vi "TestProgram1Keithley2.vi"() -> ()   [LabVIEW 2014]
panel:
  out "Resistance":dbl
  in  "Delay":dbl
  in  "Average Measurements":dbl
  in  "Clear graph?":bool
  out "Resistance VS Temperature":cluster{dbl[], dbl[]}(graph)
  out "Byte Stream File Refnum":refnum<file>
  in  "file path (use dialog)":path
  out "Current Temperature":string
  out "Return":string
  in  "Set Temperature Command":string
  in  "Set Temperature":bool
  out "Return Value Temp":string
  in  "Command Temp":string
  in  "Temp":refnum<visa-resource-name>
  in  "Multimeter 1":refnum<visa-resource-name>
  in  "Measure":bool
  in  "stop":bool
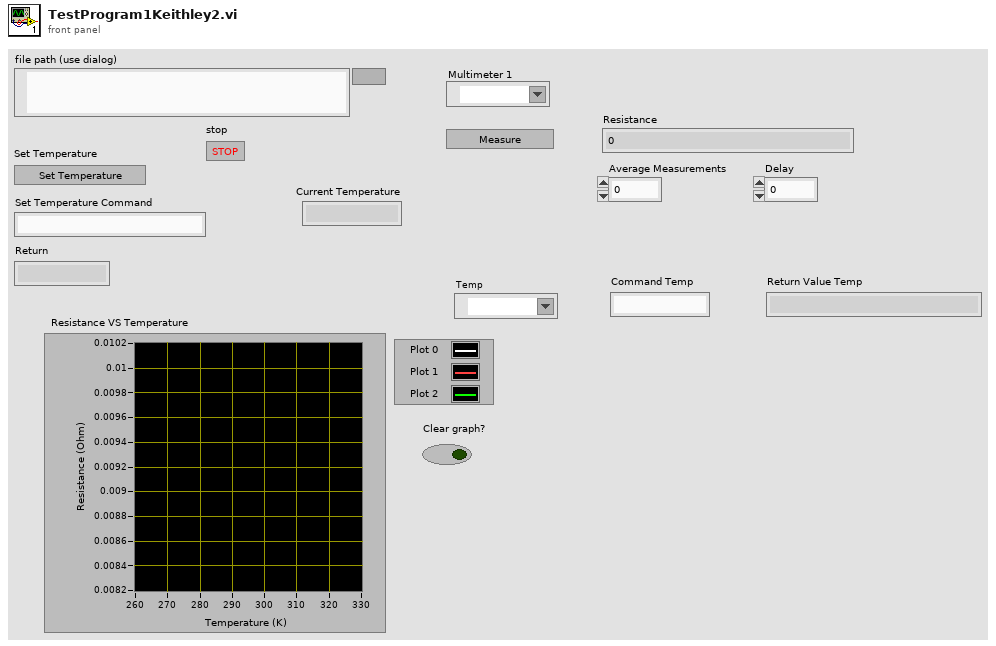
[diagram p1: front panel]
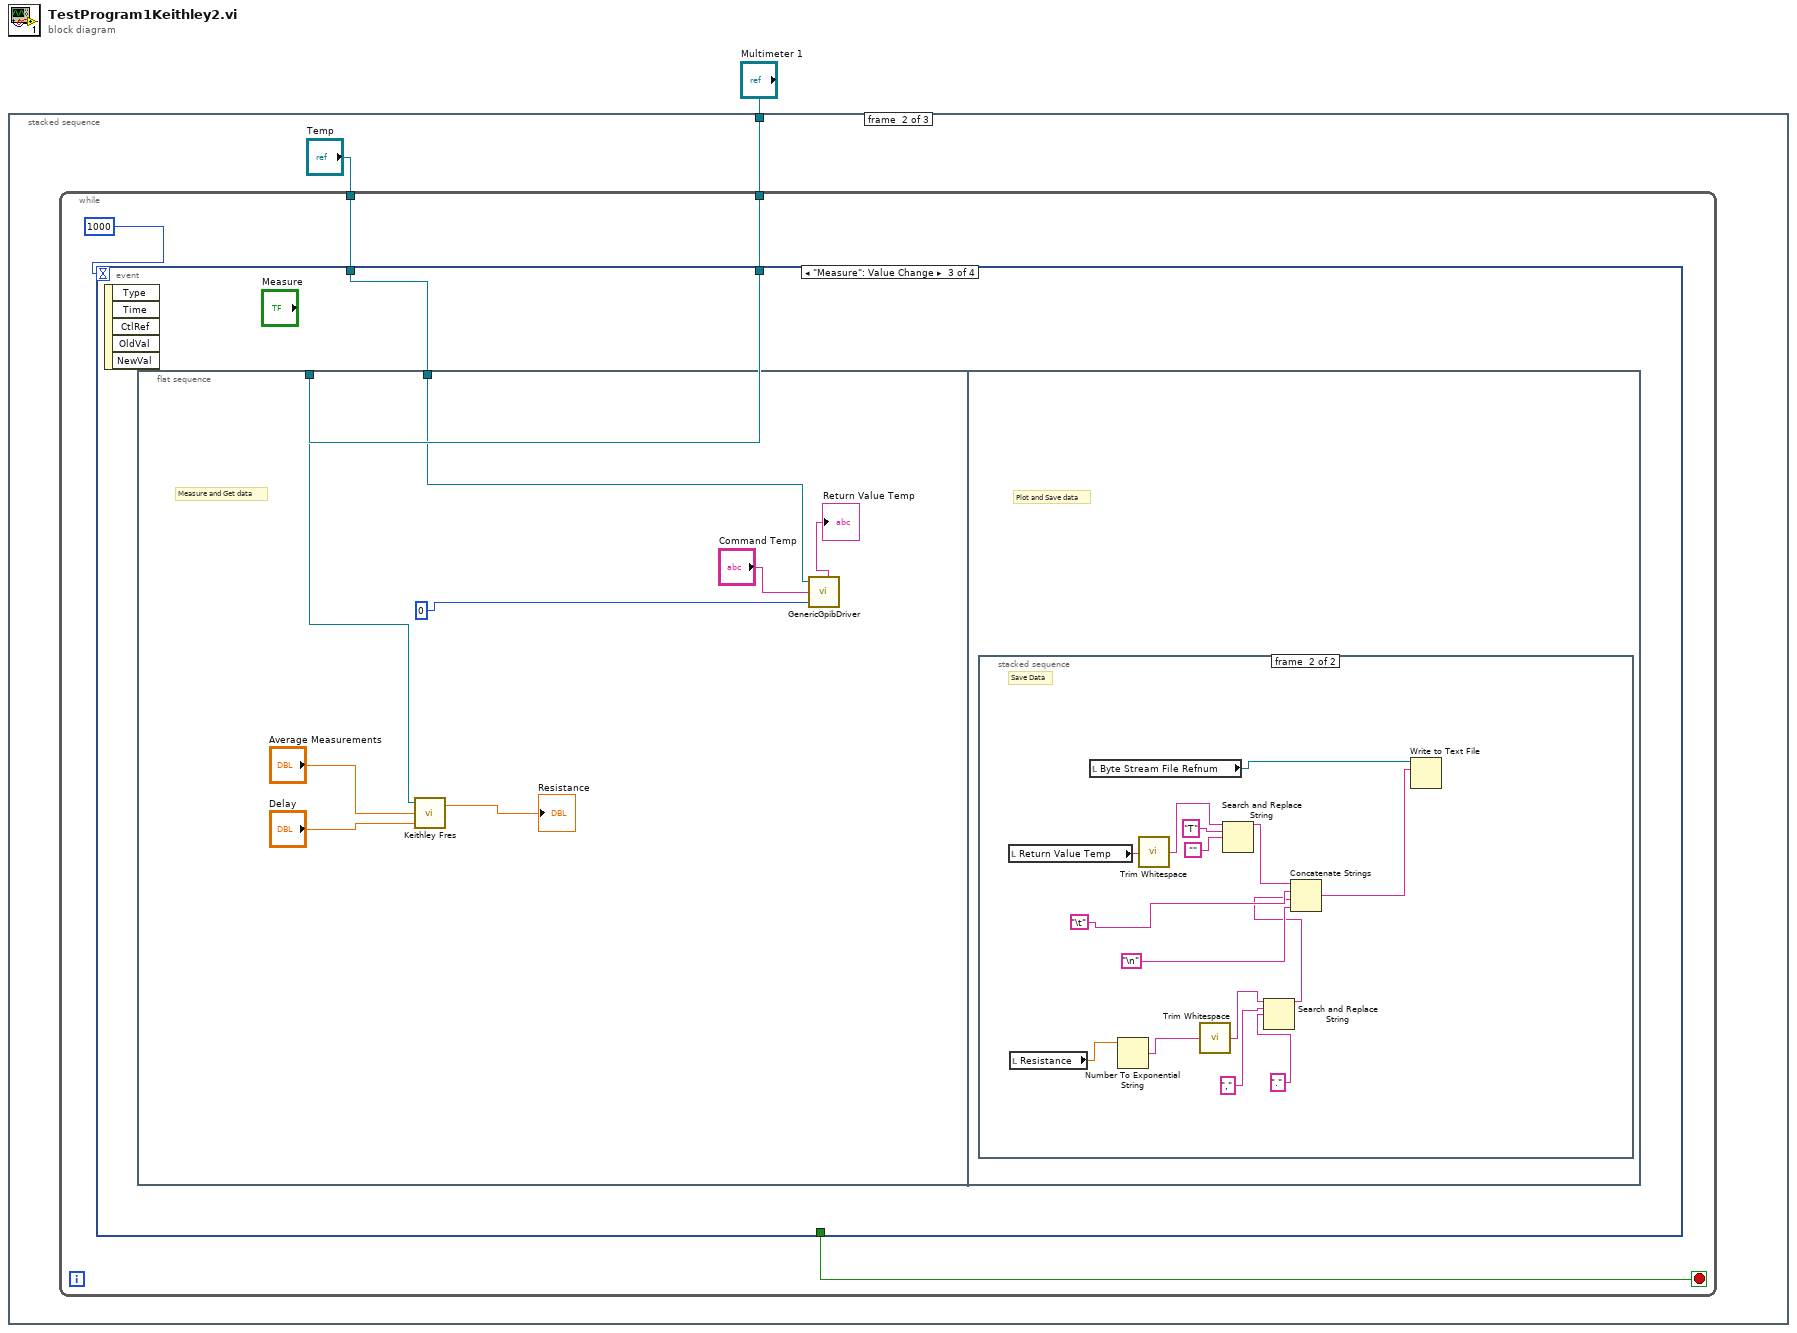
[diagram p0: block diagram]
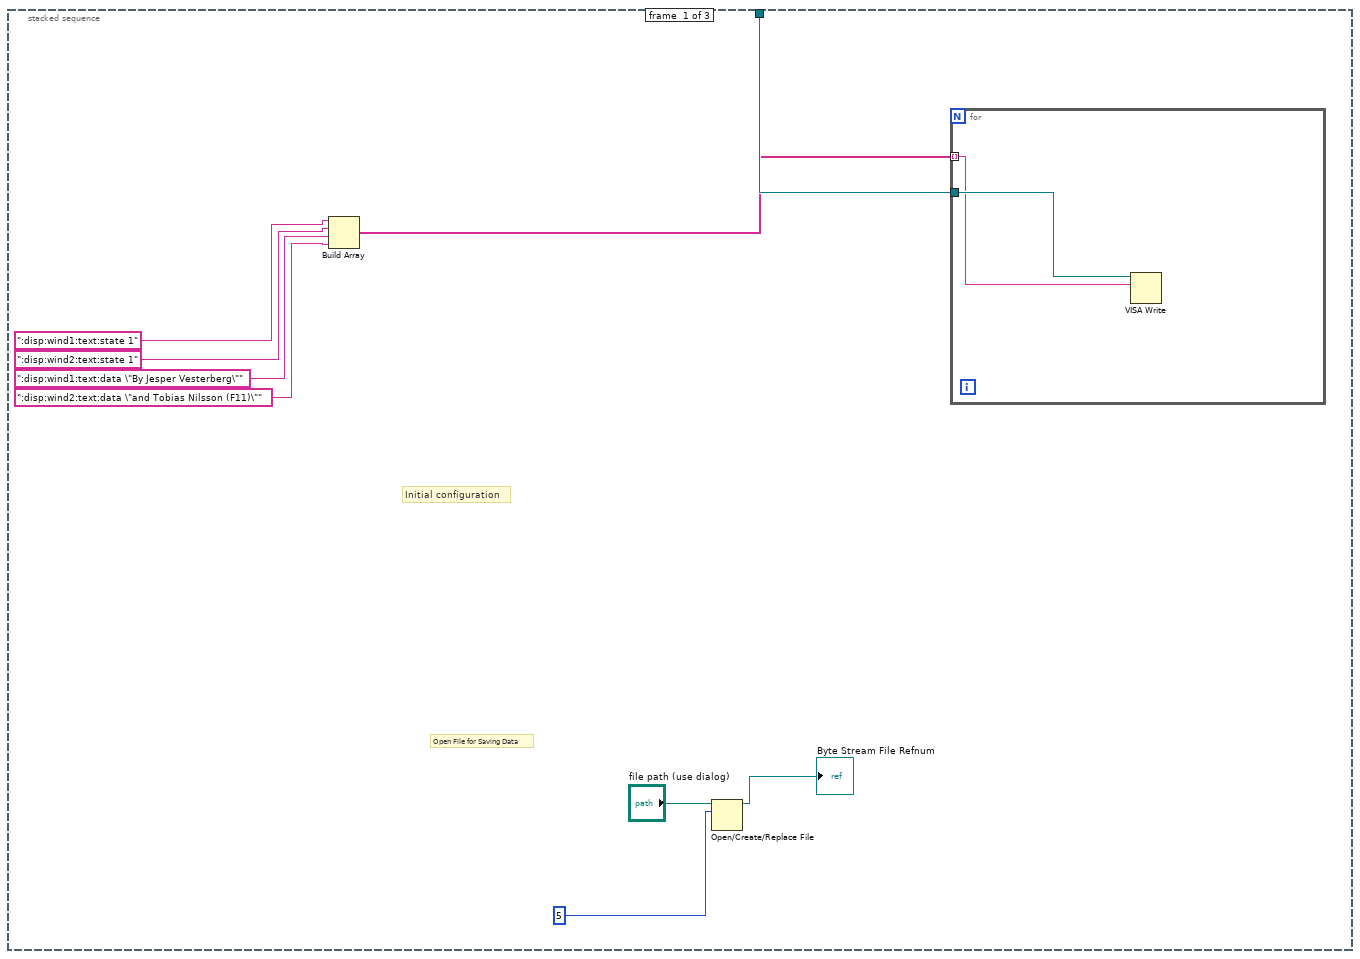
[diagram p2: hidden frame]
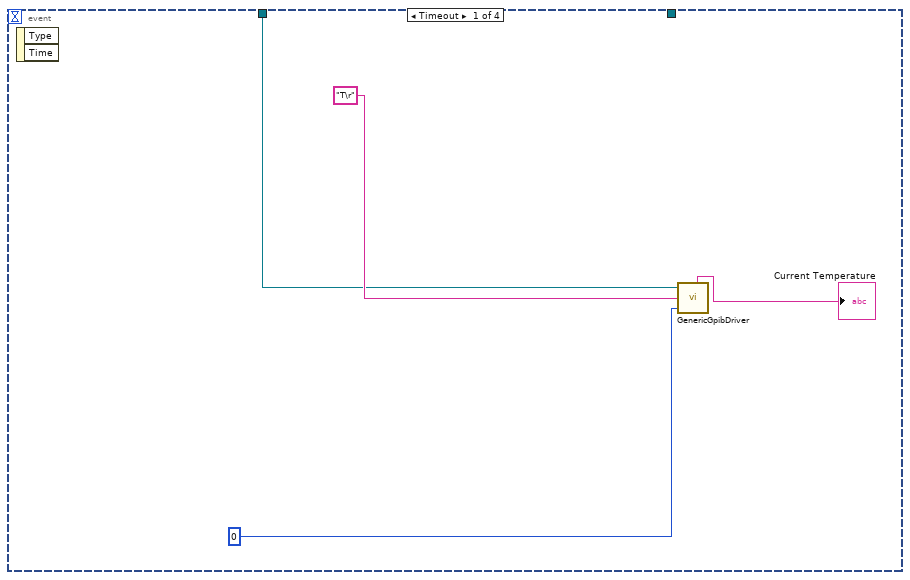
[diagram p3: hidden frame]
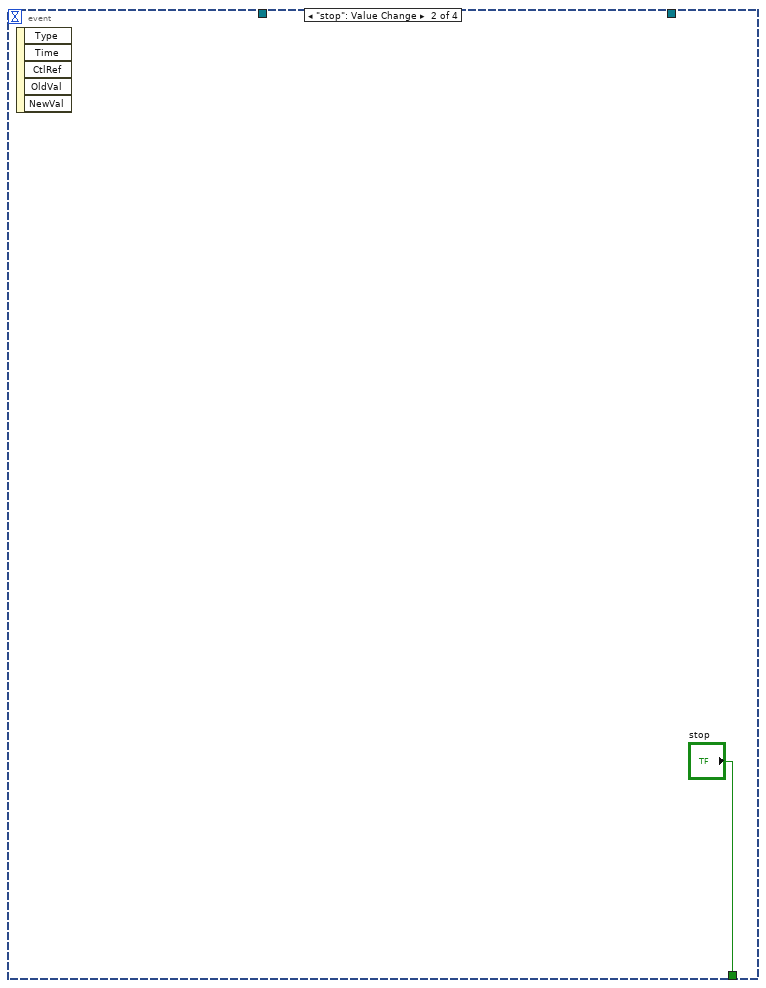
[diagram p4: hidden frame]
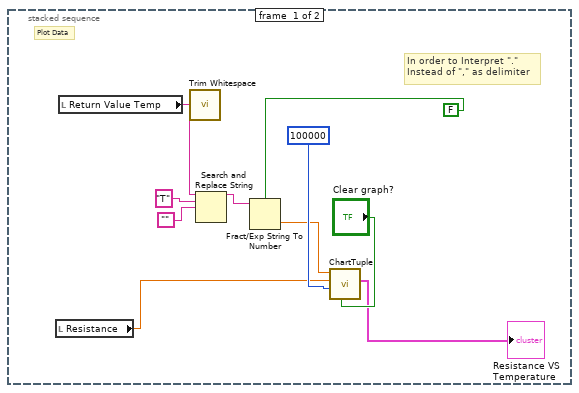
[diagram p5: hidden frame]
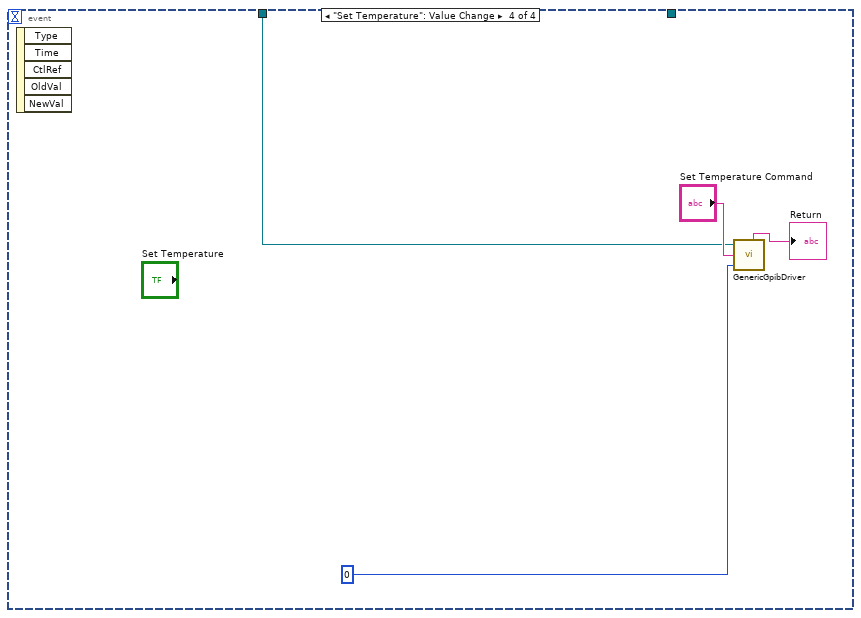
[diagram p6: hidden frame]
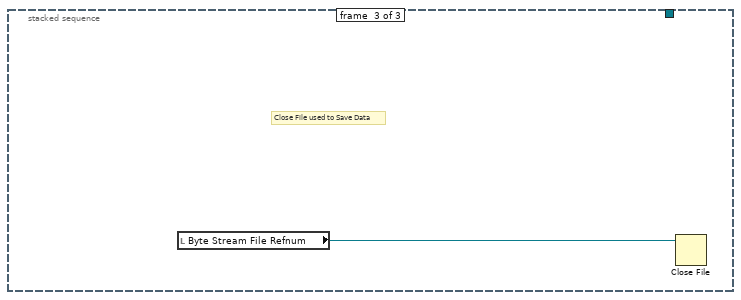
[diagram p7: hidden frame]
diagram:
  n1 = stacked-sequence {
    tunnel: "Multimeter 1" -> [w7 w13 _]
    frame #0 {
      # "Initial configuration"
      # "Open File for Saving Data"
      n2 = Build Array(":disp:wind1:text:state 1", ":disp:wind2:text:state 1", ":disp:wind1:text:data \"By Jesper Vesterberg\"", ":disp:wind2:text:data \"and Tobias Nilsson (F11)\"") -> (w6:string[])
      n3 = Open/Create/Replace File(file path (use dialog)="file path (use dialog)", operation (0:open)=5) -> (refnum out=→"Byte Stream File Refnum":refnum<file>)  [unwired: 4 in, 2 out]
      n4 = for {
        tunnel: w7 -> [w12]
        tunnel: w6 -> [w11] mode=indexing
        n5 = VISA Write(VISA resource name=w12, write buffer=w11) -> ()  [unwired: 1 in, 3 out]
      }
    }
    frame #1 {
      n6 = while {
        tunnel: "Temp" -> [w17]
        tunnel: w13 -> [w15]
        stop <- w18 stop-if-true
        n7 = event shown="[2] \"Measure\": Value Change" {
          selector: _ -> [_ _ _ _]
          dyn-events: _ -> [_ _ _ _]
          timeout: 1000 -> [_ _ _ _]
          tunnel: [_ "stop" _ _] -> w18
          tunnel: w17 -> [w21 _ w25 w61]
          tunnel: w15 -> [_ _ w24 _]
          event Timeout {
            n8 = event-data() -> ()  [unwired: 1 in, 2 out]
            n9 = call "GenericGpibDriver.vi"("Wait (ms)"=0, "Command"="T\r", "VISA resource name"=w21) -> ("Return Value"=→"Current Temperature":string)  [unwired: 1 in, 4 out]
          }
          event "stop": Value Change {
            n10 = event-data() -> ()  [unwired: 1 in, 5 out]
          }
          event "Measure": Value Change {
            n11 = event-data() -> ()  [unwired: 1 in, 5 out]
            n12 = flat-sequence {
              tunnel: w25 -> [w31]
              tunnel: w24 -> [w29]
              frame #0 {
                # "Measure and Get data"
                n13 = call "Keithley Fres.vi"("Delay"="Delay", "Average Measurements"="Average Measurements", "VISA resource name"=w29) -> ("Resistance"=→"Resistance":dbl)  [unwired: 1 in]
                n14 = call "GenericGpibDriver.vi"("Wait (ms)"=0, "Command"="Command Temp", "VISA resource name"=w31) -> ("Return Value"=→"Return Value Temp":string)  [unwired: 1 in, 4 out]
              }
              frame #1 {
                # "Plot and Save data"
                n15 = stacked-sequence {
                  frame #0 {
                    # "In order to Interpret \".\" \nInstead of \",\" as delimiter"
                    # "Plot Data"
                    n16 = local read "Resistance"() -> (w34:dbl)
                    n17 = local read "Return Value Temp"() -> (w41:string)
                    n18 = call <vilib>:"Trim Whitespace.vi"("string"=w41) -> ("trimmed string"=w40:string)  [unwired: 1 in]
                    n19 = Search and Replace String(input string=w40, search string="T", replace string="") -> (result string=w42:string)  [unwired: 5 in, 3 out]
                    n20 = Fract/Exp String To Number(use system decimal point (T)=FALSE, string=w42) -> (number=w38:dbl)  [unwired: 2 in, 1 out]
                    n21 = call "ChartTuple.vi"("Clear Graph?"="Clear graph?", "Chart History (10,000)"=100000, "Y Value"=w34, "X Value"=w38) -> ("XY Graph"=→"Resistance VS Temperature":cluster{dbl[], dbl[]})  [unwired: 7 in]
                  }
                  frame #1 {
                    # "Save Data"
                    n22 = local read "Return Value Temp"() -> (w57:string)
                    n23 = local read "Resistance"() -> (w50:dbl)
                    n24 = local read "Byte Stream File Refnum"() -> (w58:refnum<file>)
                    n25 = Number To Exponential String(number=w50) -> (E-format string=w49:string)  [unwired: 3 in]
                    n26 = call <vilib>:"Trim Whitespace.vi"("string"=w57) -> ("trimmed string"=w54:string)  [unwired: 1 in]
                    n27 = call <vilib>:"Trim Whitespace.vi"("string"=w49) -> ("trimmed string"=w48:string)  [unwired: 1 in]
                    n28 = Search and Replace String(input string=w54, search string="T", replace string="") -> (result string=w53:string)  [unwired: 5 in, 3 out]
                    n29 = Search and Replace String(input string=w48, search string=",", replace string=".") -> (result string=w45:string)  [unwired: 5 in, 3 out]
                    n30 = Concatenate Strings(w53, "\t", w45, "\n") -> (w59:string)
                    n31 = Write to Text File(file (use dialog)=w58, text=w59) -> ()  [unwired: 2 in, 3 out]
                  }
                }
              }
            }
          }
          event "Set Temperature": Value Change {
            n32 = event-data() -> ()  [unwired: 1 in, 5 out]
            n33 = call "GenericGpibDriver.vi"("Wait (ms)"=0, "Command"="Set Temperature Command", "VISA resource name"=w61) -> ("Return Value"=→"Return":string)  [unwired: 1 in, 4 out]
          }
        }
      }
    }
    frame #2 {
      # "Close File used to Save Data"
      n34 = local read "Byte Stream File Refnum"() -> (w64:refnum<file>)
      n35 = Close File(refnum=w64) -> ()  [unwired: 1 in, 2 out]
    }
  }
